vi "标定验证.vi"() -> ()   [LabVIEW 2015]
uses:
  <vilib>/vision/driver/NI_Vision_Acquisition_Software.lvlib
  <vilib>/vision/driver/IMAQdx.llb/IMAQdx Buffer Number Mode.ctl
  <vilib>/userdefined/High Color/IMAQdx.ctl
  <vilib>/vision/driver/IMAQdx.llb/IMAQdx Acquisition Mode.ctl
panel:
  in  "标定文件":string(combo)="料车1G1机种.ini"
  in  "标定坐标Y":dbl=1336.109253
  in  "标定坐标X":dbl=-857.298523
  in  "当前坐标Y":dbl
  in  "当前坐标X":dbl
  out "Image Out":T1(plugin-control)
  out "robot y":dbl
  out "robot x":dbl
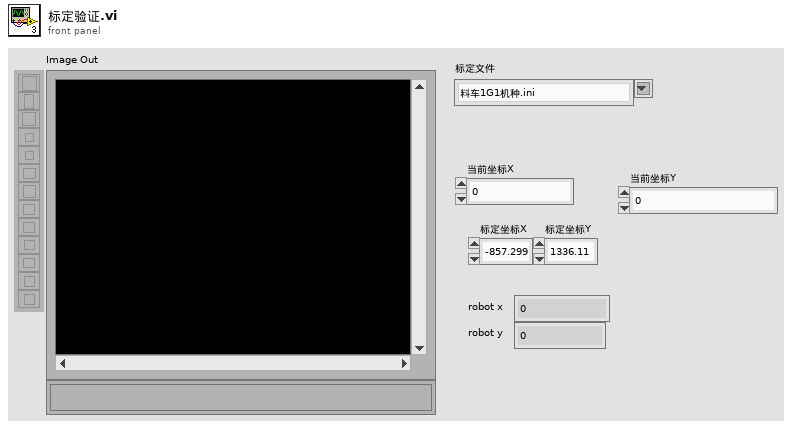
[diagram p1: front panel]
types:
  T1 = typedef "IMAQ Image.ctl" = refnum<image>
  T2 = typedef "NI_Vision_Acquisition_Software.lvlib/IMAQdx Acquisition Mode.ctl" = enum32{"One Shot", "Continuous"}
  T3 = typedef "IMAQdx.ctl" = refnum<k21>
  T4 = typedef "NI_Vision_Acquisition_Software.lvlib/IMAQdx Buffer Number Mode.ctl" = enum32{"Next", "Last", "Buffer Number", "Every", "Last New"}
  T5 = typedef "Image Type" = u32
  T6 = cluster{"Center (Pixels)":cluster{"X":sgl, "Y":sgl}, "Radius (Pixels)":dbl, "Center (Real-World)":cluster{"X":sgl, "Y":sgl}, "Radius (Real-World)":dbl, "Roundness (Real-World)":dbl, "Average Strength":dbl, "Average SNR (dB)":dbl}
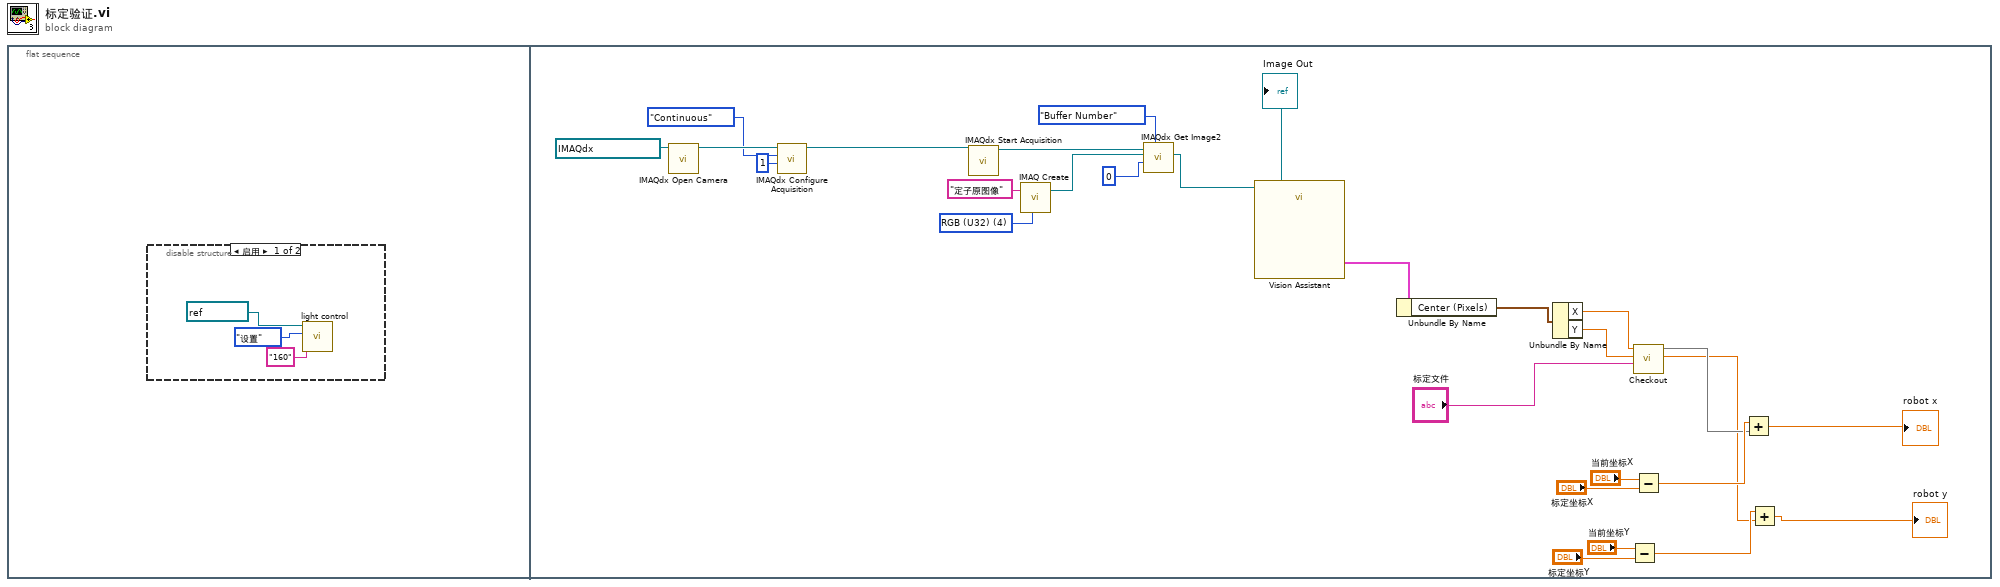
[diagram p0: block diagram]
diagram:
  n1 = flat-sequence {
    frame #0 {
      n2 = disable-structure shown="启用" {
        frame Enabled {
          n3 = call "light control.vi"("光源亮度"="160", "命令"=enum16{"打开", "设置", "关闭"}."设置", "Resource"=refnum<visa-resource-name> "COM1") -> ()  [unwired: 9 in]
        }
        frame Disabled {
        }
      }
    }
    frame #1 {
      w19 = T5 4 items=["Grayscale (U8)", "Grayscale (I16)", "Grayscale (SGL)", "Complex (CSG)", "RGB (U32)", "HSL (U32)", "RGB (U64)", "Grayscale (U16)"] ("Image Type")
      n4 = call <vilib>:"IMAQdx Open Camera.vi"("Session In"=T3 "acA1600-20gc") -> ("Session Out"=w29:T3)  [unwired: 9 in, 1 out]
      n5 = call <vilib>:"IMAQdx Configure Acquisition.vi"("Number of Buffers"=u32 1, "Continuous?"=IMAQdx_Acquisition_Mode."Continuous", "Session In"=w29) -> ("Session Out"=w21:T3)  [unwired: 7 in, 1 out]
      n6 = call <vilib>:"IMAQdx Start Acquisition.vi"("Session In"=w21) -> ("Session Out"=w22:T3)  [unwired: 9 in, 1 out]
      n7 = call "IMAQ Create"("Image Name"="定子原图像", "Image Type"=w19) -> ("New Image"=w23:T1)  [unwired: 3 in, 1 out]
      n8 = call <vilib>:"IMAQdx Get Image2.vi"("Buffer Number Mode (Next)"=IMAQdx_Buffer_Number_Mode."Buffer Number", "Buffer Number In"=u32 0, "Image In"=w23, "Session In"=w22) -> ("Image Out"=w20:T1)  [unwired: 4 in, 3 out]
      "Image Out" <- w20
      n9 = call "Vision Assistant"("Image In"=w20) -> ("Fitted Circle (Find Circular Edge 1)"=w18:T6)  [unwired: 24 in, 2 out]
      n10 = Unbundle By Name(w18) -> ("Center (Pixels)"=w17:cluster{"X":sgl, "Y":sgl})
      n11 = Unbundle By Name(w17) -> ("X"=w16:sgl, "Y"=w15:sgl)
      n12 = Subtract(x="当前坐标Y", y="标定坐标Y") -> (x-y=w9:dbl)
      n13 = call "Checkout.vi"("camera x"="标定文件", 10:w15, "Camera"=w16) -> ("robot x"=w7:dbl, 3:w8)  [unwired: 6 in, 1 out]
      n14 = Subtract(x="当前坐标X", y="标定坐标X") -> (x-y=w10:dbl)
      n15 = Add(x=w10, y=w8) -> (x+y=→"robot x":dbl)
      n16 = Add(x=w9, y=w7) -> (x+y=→"robot y":dbl)
    }
  }
